vi "SaveState.vi"(8 "error in (no error)":errorcluster, 11 "TreeControl in":refnum<vi>) -> (0 "error out":errorcluster, 2 "State":T1, 3 "TreeControl out":refnum<vi>)   [LabVIEW 2019, in "TreeControlLib.lvlib"]
uses:
  TreeControlLib.lvlib
  <vilib>/Utility/Data Type/NI_Data Type.lvlib
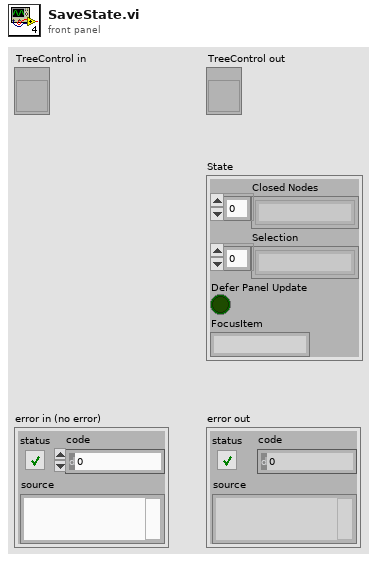
[diagram p1: front panel]
types:
  T1 = cluster{"Closed Nodes":string[], "Selection":string[], "Defer Panel Update":bool, "FocusItem":string}
  T2 = typedef "NI_Data Type.lvlib/Data Type.ctl" = enum8{"Invalid Type", "Void", "I8", "I16", "I32", "I64", "U8", "U16", "U32", "U64", "Single Float", "Double Float", "Extended Float", "Single Complex", "Double Complex", "Extended Complex", "Enum U8", "Enum U16", "Enum U32", "Enum U64", "Single Float With Unit", "Double Float With Unit", "Extended Float With Unit", "Single Complex with Unit", "Double Complex with Unit", "Extended Complex with Unit", "Boolean", "String", "Path", "Picture", "Tag", "Array", "Cluster", "Variant", "LV Variant", "Waveform", "Timestamp", "Digital Waveform", "Digital Data", "ExpressData", "Refnum", "External Data", "VI", "Poly VI", "LabVIEW Class Instance", "Fixed Point", "Set Collection", "Map Collection"}
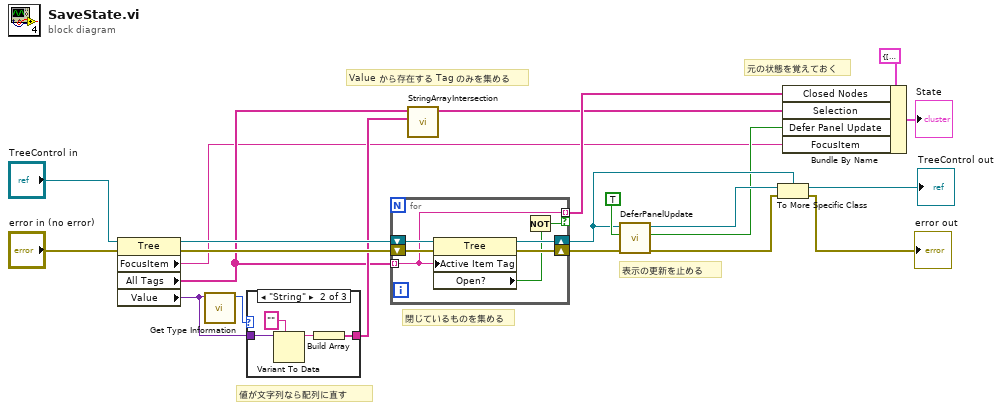
[diagram p0: block diagram]
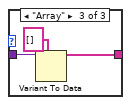
[diagram p3: hidden frame]
diagram:
  # "値が文字列なら配列に直す"
  # "元の状態を覚えておく"
  # "表示の更新を止める"
  # "Value から存在する Tag のみを集める"
  # "閉じているものを集める"
  n1 = property class="Tree"(reference="TreeControl in", error in="error in (no error)") -> (reference out=w20:refnum<vi>, error out=w21:errorcluster, "FocusItem"=w2:string, "All Tags"=w3:string[], "Value"=w6:variant)
  n2 = call <vilib>:"Get Type Information.vi"("variant"=w6) -> ("type"=w7:T2)  [unwired: 6 in, 4 out]
  n3 = case shown="\"String\"" w7 {
    tunnel: w6 -> [_ w25 w28]
    tunnel: [_ w22 w26] -> w5
    frame Default {
    }
    frame "String" {
      n4 = Variant To Data(type="", Variant=w25) -> (data=w23:string)  [unwired: 1 in, 1 out]
      n5 = Build Array(w23) -> (w22:string[])
    }
    frame "Array" {
      n6 = Variant To Data(type=string[] [], Variant=w28) -> (data=w26:string[])  [unwired: 1 in, 1 out]
    }
  }
  n7 = for {
    tunnel: w3 -> [w31] mode=indexing
    shift-right: [w33] -> w14
    shift-left: w20 -> [w35]
    shift-right: [w32] -> w15
    shift-left: w21 -> [w34]
    tunnel: [w31] -> w11 mode=indexing if=w29
    n8 = property class="Tree"(reference=w35, error in=w34, "Active Item Tag"=w31) -> (reference out=w33:refnum<vi>, error out=w32:errorcluster, "Open?"=w30:bool)
    n9 = Not(x=w30) -> (.not. x?=w29:bool)
  }
  n10 = call "StringArrayIntersection.vi"("Fewer"=w5, "More"=w3) -> ("Intersection"=w10:string[])  [unwired: 9 in]
  n11 = call "DeferPanelUpdate.vi"("error in (no error)"=w15, "Defer Panel Updates (T)"=TRUE ("Defer Panel Updates"), "Control in"=w14) -> ("error out"=w9:errorcluster, "Defer Panel Updates Old"=w12:bool, "Control out"=w17:refnum<vi>)  [unwired: 6 in]
  n12 = To More Specific Class(target class=w14, reference=w17, error in=w9) -> (specific class reference=→"TreeControl out":refnum<vi>, error out=→"error out":errorcluster)
  n13 = Bundle By Name(cluster=T1 {"Closed Nodes"=[], "Selection"=[], "Defer Panel Update"=TRUE, "FocusItem"=""} ("Cluster"), "Closed Nodes"=w11, "Selection"=w10, "Defer Panel Update"=w12, "FocusItem"=w2) -> (→"State":T1)
